vi "Immediate Surroundings.vi"(9 "Direction":T1, 10 "Column":i32, 11 "Row":i32) -> (2 "Columns":i32[](array[numeric]), 3 "Rows":i32[](array[numeric]))   [LabVIEW 2015, in "Defenders.lvclass"]
uses:
  Defenders.lvclass
  Type Defs/Direction Enum.ctl
  SubVIs/Read-Only Globals.vi
  SubVIs/Globals (private).vi
  Square/Square.lvclass
  Type Defs/SB Type Defs.lvlib
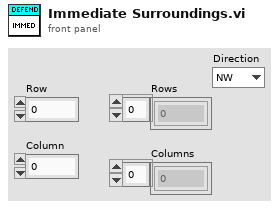
[diagram p1: front panel]
types:
  T1 = typedef "SB Type Defs.lvlib/Direction Enum.ctl" = enum16{"NW", "N", "NE", "E", "SE", "S", "SW", "W"}
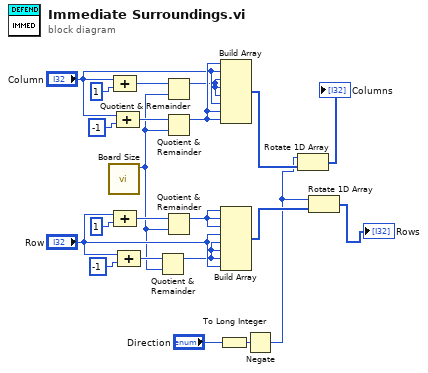
[diagram p0: block diagram]
diagram:
  n1 = call "Board Size.vi"() -> ("Board Size"=w1:i32)  [unwired: 11 in]
  n2 = Compound Arithmetic op=ADD("Column", 1 ("value")) -> (w16:i32)
  n3 = Compound Arithmetic op=ADD("Row", 1 ("value")) -> (w13:i32)
  n4 = Compound Arithmetic op=ADD("Column", -1 ("value")) -> (w20:i32)
  n5 = Compound Arithmetic op=ADD("Row", -1 ("value")) -> (w3:i32)
  n6 = Quotient & Remainder(x=w3, y=w1) -> (x-y*floor(x/y)=w2:i32)  [unwired: 1 out]
  n7 = Quotient & Remainder(x=w16, y=w1) -> (x-y*floor(x/y)=w15:i32)  [unwired: 1 out]
  n8 = Quotient & Remainder(x=w20, y=w1) -> (x-y*floor(x/y)=w19:i32)  [unwired: 1 out]
  n9 = Quotient & Remainder(x=w13, y=w1) -> (x-y*floor(x/y)=w14:i32)  [unwired: 1 out]
  n10 = To Long Integer(number="Direction") -> (32bit integer=w5:i32)
  n11 = Build Array(w19, "Column", w15, w15, w15, "Column", w19, w19) -> (w10:i32[])
  n12 = Build Array(w14, w14, w14, "Row", w2, w2, w2, "Row") -> (w7:i32[])
  n13 = Negate(x=w5) -> (-x=w4:i32)
  n14 = Rotate 1D Array(1:w10, 2:w4) -> (0:→"Columns":i32[])
  n15 = Rotate 1D Array(1:w7, 2:w4) -> (0:→"Rows":i32[])
